vi "Main.vi"(10 "Mensajes Sub panel":refnum<vi>, 11 "Module Admin":refnum<class "Delacor_lib_QMH_Module Admin.lvclass">) -> ()   [LabVIEW 2019, in "Analisis.lvlib"]
doc: "This template is based off of the Queued Message Handler design pattern and the Queued Message Handler project template that ships with LabVIEW.\n\nThe main difference is that the queue is private to this module and communication between modules is performed via Broadcast and Request events.\n\nRequest events are wrapped in public API methods and are handled in the Event Handling Loop (EHL) of this VI. Any module can register for Broadcast events sent by this module. The EHL generates messages based on user interface actions.\n\nThe Message Handling Loop (MHL) processes messages generated by the EHL, or by other messages. The messages are string values, so new messages can be added easily to the Message Cases case structure in the MHL. Each message cluster can also provide an optional value for Message Data, which is a variant that can be converted to whatever message-specific data is required.\n_____\nBased on Delacor QMH Project Template 5.0.0.82.\n\nAnalisis\n\nEste modulo es similar a el de adquisicion y base de datos, solamente que aqui ciclamos el analisis de la imagen por medio de un VI generado desde vission assistant, en el cual analisamos, la forma de una marca, el color de la tarjeta y el nombre del indivduo, al igual que los otros modulos cuenta con un helper loop y eventos de configuracion."
uses:
  Analisis.lvlib
  <vilib>/Delacor/Delacor QMH/Libraries/Module Admin_class/Delacor_lib_QMH_Module Admin.lvclass
  Module Data--cluster.ctl
  Iniciar analisis Argument--cluster.ctl
  Parar Analisis Argument--cluster.ctl
  <vilib>/vision/Image Controls.llb/IMAQ Image.ctl
  Analisis de imagenes Argument--cluster.ctl
  Stop Argument--cluster.ctl
  <vilib>/Delacor/Delacor QMH/Libraries/Message Queue_class/Delacor_lib_QMH_Message Queue.lvclass/Delacor_lib_QMH_Message Queue.ctl
  <vilib>/Delacor/Delacor QMH/Libraries/Module Admin_class/Delacor_lib_QMH_Module Admin.lvclass/Delacor_lib_QMH_Module Admin.ctl
  <vilib>/Utility/miscctls.llb/LVPointTypeDef.ctl
  <vilib>/Delacor/Delacor QMH/Libraries/Message Queue_class/Delacor_lib_QMH_Enqueue Message (Single).vi
  <vilib>/Delacor/Delacor QMH/Libraries/Module Admin_class/Delacor_lib_QMH_Get External Launch.vi
  <vilib>/Utility/error.llb/Error Cluster From Error Code.vi
  <vilib>/ErrorRing/Error Ring.xnode
  <vilib>/Delacor/Delacor QMH/Libraries/Message Queue_class/Delacor_lib_QMH_Message Queue.lvclass
  Base de datos/Base de datos.lvlib
panel:
  out "Hora de Entrada":timestamp
  out "Area":string
  out "Nombre":string
  out "Empresa":string
  out "error out":errorcluster
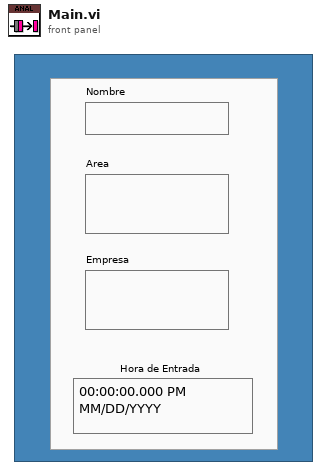
[diagram p1: front panel]
types:
  T1 = typedef "Analisis.lvlib/Request Events--cluster.ctl" = cluster{"Stop Module":refnum<user-event>, "Show Panel":refnum<user-event>, "Hide Panel":refnum<user-event>, "Get Module Execution Status":refnum<user-event>, "Show Diagram":refnum<user-event>, "Iniciar analisis":refnum<user-event>, "Parar Analisis":refnum<user-event>, "Analisis de imagenes":refnum<user-event>}
  T2 = typedef "Analisis.lvlib/Module Data--cluster.ctl" = cluster{"Status":string}
  T3 = typedef "IMAQ Image.ctl" = refnum<image>
  T4 = typedef "Analisis.lvlib/Parar Analisis Argument--cluster.ctl" = cluster{"Boolean":bool}
  T5 = typedef "Analisis.lvlib/Analisis de imagenes Argument--cluster.ctl" = cluster{"New Image":T3}
  T6 = enum32{"invalid lock state", "Not Locked", "Locked (No Password)", "Password-protected"}
  T7 = typedef "Analisis.lvlib/Stop Argument--cluster.ctl" = cluster{"Origin":string, "Exit via Stop Module Req?":bool, "Wait for Module to stop?":bool}
  T8 = typedef "LVPointTypeDef.ctl" = cluster{"Horizontal":i16, "Vertical":i16}
  T9 = enum32{"Invalid", "Standard", "Closed", "Hidden", "Minimized", "Maximized"}
  T10 = typedef "Image Type" = u32
  T11 = typedef "Analisis.lvlib/Iniciar analisis Argument--cluster.ctl" = cluster{"Boolean":bool}
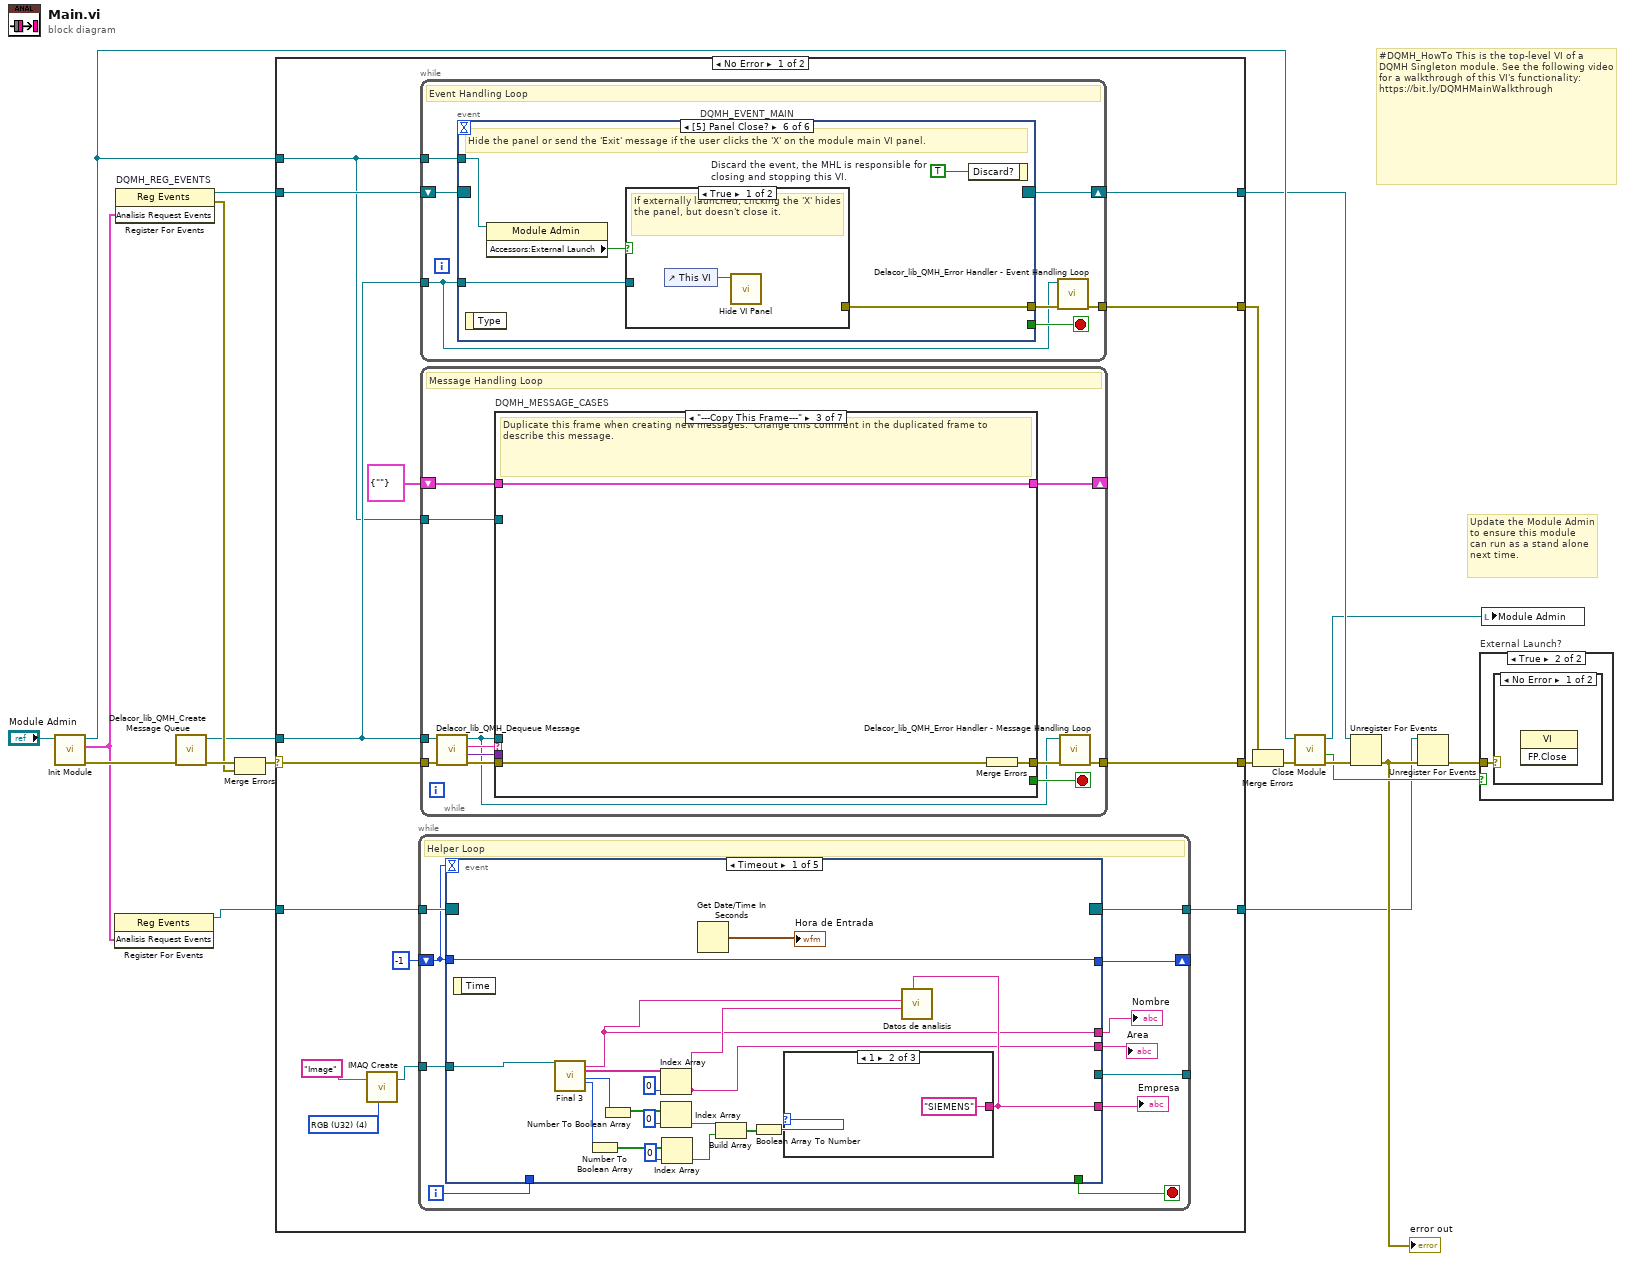
[diagram p0: block diagram]
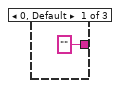
[diagram p2: hidden frame]
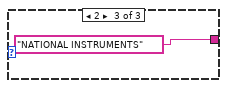
[diagram p3: hidden frame]
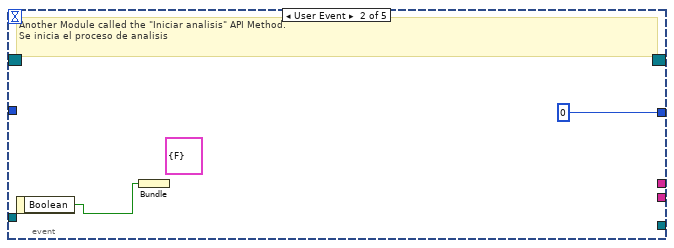
[diagram p4: hidden frame]
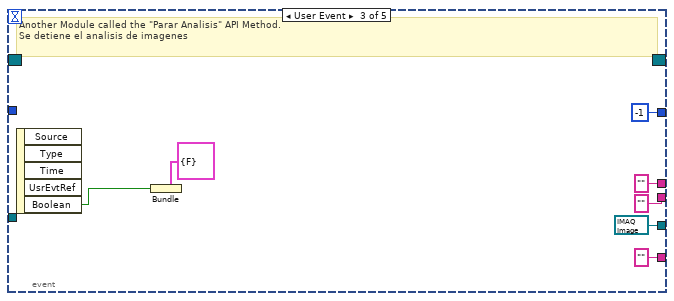
[diagram p5: hidden frame]
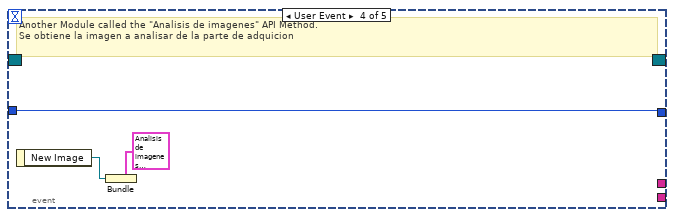
[diagram p6: hidden frame]
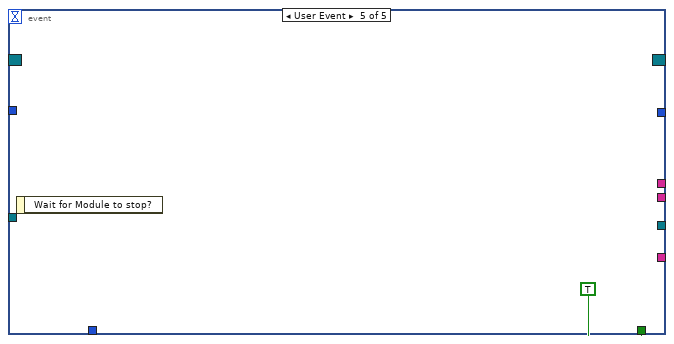
[diagram p7: hidden frame]
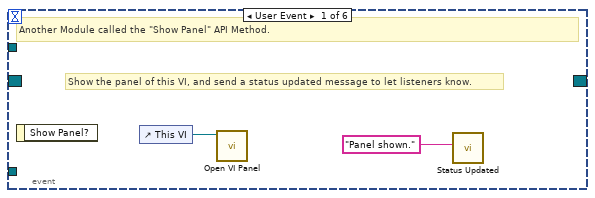
[diagram p8: hidden frame]
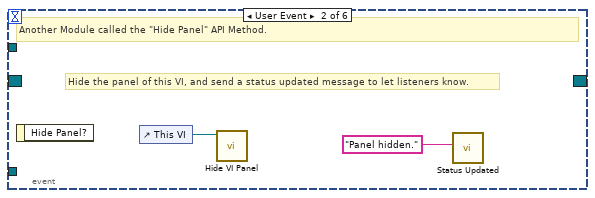
[diagram p9: hidden frame]
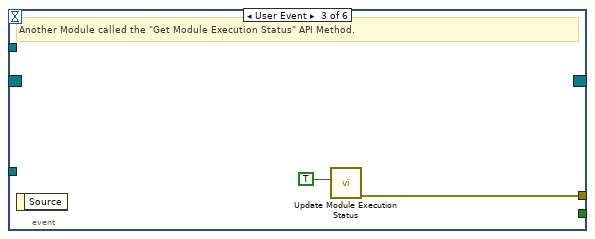
[diagram p10: hidden frame]
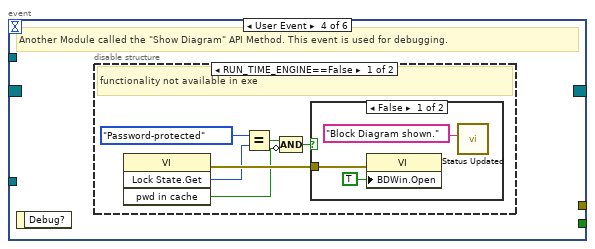
[diagram p11: hidden frame]
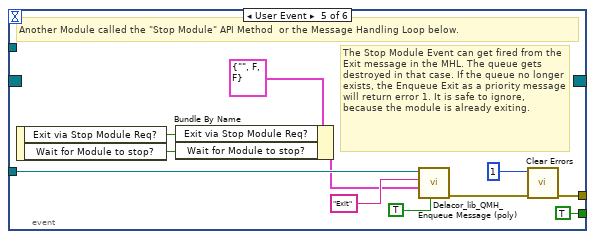
[diagram p14: hidden frame]
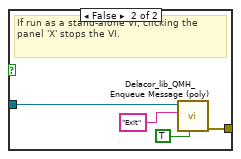
[diagram p15: hidden frame]
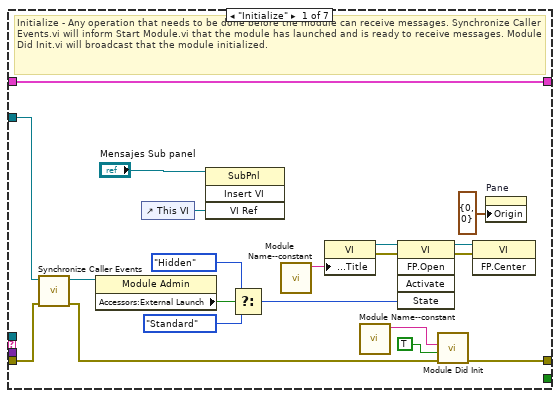
[diagram p16: hidden frame]
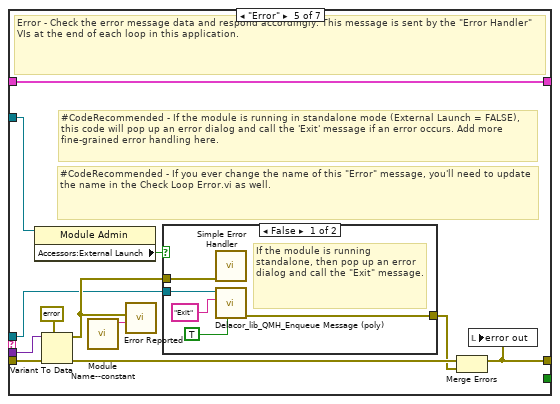
[diagram p19: hidden frame]
diagram:
  # "#DQMH_HowTo This is the top-level VI of a DQMH Singleton module. See the following video for a walkthrough of this VI's functionality: https://bit.ly/DQMHMainWalkthrough"
  # "Update the Module Admin to ensure this module can run as a stand alone next time."
  n1 = call "Init Module.vi"("Singleton Module Admin in"="Module Admin") -> ("error out"=w19:errorcluster, "Analisis Request Events"=w5:T1, "Singleton Module Admin out"=w12:refnum<class "Delacor_lib_QMH_Module Admin.lvclass">)  [unwired: 8 in]
  n2 = register-events(w5) -> (reference out=w4:refnum<event-registration>)  [unwired: 2 in, 1 out]
  n3 = register-events "DQMH_REG_EVENTS"(w5) -> (reference out=w10:refnum<event-registration>, error out=w13:errorcluster)  [unwired: 2 in]
  n4 = call <vilib>:"Delacor_lib_QMH_Create Message Queue.vi"("error in (no error)"=w19) -> ("error out"=w15:errorcluster, "Message Queue"=w9:refnum<class "Delacor_lib_QMH_Message Queue.lvclass">)  [unwired: 9 in]
  n5 = Merge Errors(w15, w13) -> (w14:errorcluster)
  n6 = case shown="No Error" w14 {
    selector: w14 -> [w32 w211]
    tunnel: [w34 w210] -> w20
    tunnel: [w31 w216] -> w11
    tunnel: w10 -> [w29 w216]
    tunnel: w9 -> [w28 w209]
    tunnel: [w33 _] -> w17
    tunnel: w12 -> [w27 w212]
    tunnel: w4 -> [w26 w208]
    tunnel: [w25 w208] -> w1
    frame No Error {
      w22 = T10 4 items=["Grayscale (U8)", "Grayscale (I16)", "Grayscale (SGL)", "Complex (CSG)", "RGB (U32)", "HSL (U32)", "RGB (U64)", "Grayscale (U16)"] ("Image Type")
      n7 = call "IMAQ Create"("Image Name"="Image", "Image Type"=w22) -> ("New Image"=w21:T3)  [unwired: 3 in, 1 out]
      n8 = while {
        tunnel: w26 -> [w45]
        tunnel: [w44] -> w25
        shift-right: [w42] -> _
        shift-left: -1 -> [w41]
        tunnel: [w40] -> _
        tunnel: w21 -> [w39]
        i -> [w38]
        stop <- w43 stop-if-true
        # "Helper Loop"
        n9 = event shown="[0] Timeout" {
          selector: w45 -> [_ _ _ _ _]
          dyn-events: [_ _ _ _ _] -> w44
          timeout: w41 -> [_ _ _ _ _]
          tunnel: [_ _ _ _ TRUE] -> w43
          tunnel: [w63 0 -1 w76 _] -> w42
          tunnel: w41 -> [w63 _ _ w76 _]
          tunnel: [_ _ T3 refnum ("New Image") _ _] -> w40
          tunnel: w39 -> [w62 _ _ _ _]
          tunnel: w38 -> [_ _ _ _ _]
          tunnel: [w49 _ "" ("String 4") _ _] -> w35
          tunnel: [w48 _ "" ("Class") _ _] -> w36
          tunnel: [w47 _ "" ("String (OCR/OCV 1)") _ _] -> w37
          event Timeout {
            n10 = event-data() -> ()  [unwired: 1 in, 1 out]
            n11 = call "Final 3.vi"("Image In"=w62) -> ("String (OCR/OCV 1)"=w47:string, "Classes (Color Classification 1)"=w61:string[], "Number of Matches (Color Location 1)"=w59:i32, "Number of Matches (Color Location 2)"=w58:i32)  [unwired: 20 in, 3 out]
            n12 = Number To Boolean Array(number=w58) -> (Boolean array=w54:bool[])
            n13 = Number To Boolean Array(number=w59) -> (Boolean array=w55:bool[])
            n14 = Index Array(array=w61, index=0) -> (element=w48:string)
            n15 = Index Array(array=w55, index=0) -> (element=w53:bool)
            n16 = Index Array(array=w54, index=0) -> (element=w52:bool)
            n17 = Get Date/Time In Seconds() -> (seconds since 1Jan1904=→"Hora de Entrada":timestamp)
            n18 = Build Array(w53, w52) -> (w51:bool[])
            n19 = Boolean Array To Number(Boolean array=w51) -> (number=w50:u32)
            n20 = case shown="1" w50 {
              tunnel: ["" ("String 4") "SIEMENS" ("String 4") "NATIONAL INSTRUMENTS" ("String 4")] -> w49
              frame 0, Default {
              }
              frame 1 {
              }
              frame 2 {
              }
            }
            n21 = call "Datos de analisis.vi"("String 3"=w49, "String 2"=w48, "String"=w47) -> ()  [unwired: 8 in, 1 out]
          }
          event User Event {
            (unwired) T11 {"Boolean"=FALSE} ("Iniciar analisis Argument")
            # "Another Module called the \"Iniciar analisis\" API Method.\nSe inicia el proceso de analisis"
            n22 = event-data() -> ("Boolean"=w68:bool)  [unwired: 1 in]
            n23 = Bundle("Boolean"=w68) -> ()  [unwired: 1 in, 1 out]
          }
          event User Event {
            # "Another Module called the \"Parar Analisis\" API Method.\nSe detiene el analisis de imagenes"
            n24 = event-data() -> ("Boolean"=w74:bool)  [unwired: 1 in, 4 out]
            n25 = Bundle(cluster=T4 {"Boolean"=FALSE} ("Parar Analisis Argument"), "Boolean"=w74) -> ()  [unwired: 1 out]
          }
          event User Event {
            # "Another Module called the \"Analisis de imagenes\" API Method.\nSe obtiene la imagen a analisar de la parte de adquicion"
            n26 = event-data() -> ("New Image"=w77:T3)  [unwired: 1 in]
            n27 = Bundle(cluster=T5 {"New Image"=refnum} ("Analisis de imagenes Argument"), "New Image"=w77) -> ()  [unwired: 1 out]
          }
          event User Event {
            n28 = event-data() -> ()  [unwired: 1 in, 1 out]
          }
        }
        "Area" <- w36
        "Nombre" <- w37
        "Empresa" <- w35
      }
      n29 = while {
        tunnel: w28 -> [w80]
        shift-right: [w83] -> w31
        shift-left: w29 -> [w84]
        tunnel: [w85] -> w33
        tunnel: w27 -> [w81]
        stop <- w82 stop-if-true
        # "Event Handling Loop"
        n30 = event "DQMH_EVENT_MAIN" shown="[5] Panel Close?" {
          selector: w84 -> [_ _ _ _ _ _]
          dyn-events: [_ _ _ _ _ _] -> w83
          timeout: _ -> [_ _ _ _ _ _]
          tunnel: [_ _ _ _ TRUE ("Discard?") _] -> w82
          tunnel: w80 -> [_ _ _ _ w108 w115]
          tunnel: [_ _ w92 _ w111 w117] -> w86
          tunnel: w81 -> [_ _ _ _ _ w114]
          event User Event {
            # "Show the panel of this VI, and send a status updated message to let listeners know."
            # "Another Module called the \"Show Panel\" API Method."
            n31 = event-data() -> ()  [unwired: 1 in, 1 out]
            n32 = control-ref of="This VI"() -> (w88:refnum<vi>)
            n33 = call "Open VI Panel.vi"("VI"=w88) -> ()  [unwired: 10 in, 1 out]
            n34 = call "Status Updated.vi"("Status"="Panel shown." ("format string")) -> ()  [unwired: 10 in, 1 out]
          }
          event User Event {
            # "Hide the panel of this VI, and send a status updated message to let listeners know."
            # "Another Module called the \"Hide Panel\" API Method."
            n35 = event-data() -> ()  [unwired: 1 in, 1 out]
            n36 = control-ref of="This VI"() -> (w90:refnum<vi>)
            n37 = call "Hide VI Panel.vi"("VI"=w90) -> ()  [unwired: 10 in, 1 out]
            n38 = call "Status Updated.vi"("Status"="Panel hidden." ("format string")) -> ()  [unwired: 10 in, 1 out]
          }
          event User Event {
            # "Another Module called the \"Get Module Execution Status\" API Method."
            n39 = event-data() -> ()  [unwired: 1 in, 1 out]
            n40 = call "Update Module Execution Status.vi"("Running?"=TRUE) -> ("error out"=w92:errorcluster)  [unwired: 10 in]
          }
          event User Event {
            # "Another Module called the \"Show Diagram\" API Method. This event is used for debugging."
            n41 = event-data() -> ()  [unwired: 1 in, 1 out]
            n42 = disable-structure shown="RUN_TIME_ENGINE==False" {
              frame condition #0 (active) {
                # "functionality not available in exe"
                n43 = invoke class="VI" method="Lock State.Get"() -> (error out=w98:errorcluster, "Get Lock State"=w97:T6, "pwd in cache"=w94:bool)  [unwired: 4 in, 1 out]
                n44 = Equal?(x=T6."Password-protected", y=w97) -> (x = y?=w95:bool)
                n45 = Compound Arithmetic op=AND(w95, invert w94) -> (w93:bool)
                n46 = case shown="False" w93 {
                  tunnel: w98 -> [w101 _]
                  frame False {
                    n47 = property class="VI"(error in=w101, "BDWin.Open"=TRUE ("Block Diagram Window:Open")) -> ()  [unwired: 1 in, 2 out]
                    n48 = call "Status Updated.vi"("Status"="Block Diagram shown." ("format string")) -> ()  [unwired: 10 in, 1 out]
                  }
                  frame True {
                    # "Password-protected VI, and the password is not in the cache. Do not show the diagram."
                  }
                }
              }
              frame condition #1 {
              }
            }
          }
          event User Event {
            # "The Stop Module Event can get fired from the Exit message in the MHL. The queue gets destroyed in that case. If the queue no longer exists, the Enqueue Exit as a priority message will return error 1. It is safe to ignore, because the module is already exiting."
            # "Another Module called the \"Stop Module\" API Method  or the Message Handling Loop below."
            n49 = event-data() -> ("Exit via Stop Module Req?"=w104:bool, "Wait for Module to stop?"=w103:bool)  [unwired: 1 in]
            n50 = Bundle By Name(cluster=T7 {"Origin"="", "Exit via Stop Module Req?"=FALSE, "Wait for Module to stop?"=FALSE} ("Stop Argument"), "Exit via Stop Module Req?"=w104, "Wait for Module to stop?"=w103) -> (w102:T7)
            n51 = call-poly <vilib>:"Delacor_lib_QMH_Enqueue Message (poly).vi"("Priority Message? (F)"=TRUE, "Message Data"=w102, "Message"="Exit", "Message Queue in"=w108) -> ("error out"=w112:errorcluster)  [unwired: 6 in, 1 out]
            n52 = call <vilib>:"Clear Errors.vi"("error in (no error)"=w112, "specific error code to clear (0: all)"=1) -> ("error out"=w111:errorcluster)  [unwired: 4 in, 1 out]
          }
          event Panel Close? {
            w116 = TRUE  # Discard the event, the MHL is responsible for closing and stopping this VI.
            # "Hide the panel or send the 'Exit' message if the user clicks the 'X' on the module main VI panel."
            n53 = event-data() -> ()  [unwired: 1 in, 1 out]
            n54 = property class="Module Admin"(reference=w114) -> ("Accessors:External Launch"=w113:bool)  [unwired: 1 in, 2 out]
            n55 = case shown="True" w113 {
              tunnel: w115 -> [_ w121]
              tunnel: [_ w122] -> w117
              frame True {
                # "If externally launched, clicking the 'X' hides the panel, but doesn't close it."
                n56 = control-ref of="This VI"() -> (w118:refnum<vi>)
                n57 = call "Hide VI Panel.vi"("VI"=w118) -> ()  [unwired: 10 in, 1 out]
              }
              frame False {
                # "If run as a stand-alone VI, clicking the panel 'X' stops the VI."
                n58 = call-poly <vilib>:"Delacor_lib_QMH_Enqueue Message (poly).vi"("Priority Message? (F)"=TRUE, "Message"="Exit", "Message Queue in"=w121) -> ("error out"=w122:errorcluster)  [unwired: 7 in, 1 out]
              }
            }
            n59 = event-data("Discard?"=w116) -> ()  [unwired: 1 in, 1 out]
          }
        }
        n60 = call-dynamic "Delacor_lib_QMH_Error Handler - Event Handling Loop.vi"("error in (no error)"=w86, "Message Queue in"=w80) -> ("dup error in"=w85:errorcluster)  [unwired: 8 in, 1 out]
      }
      n61 = while {
        tunnel: w28 -> [w125]
        shift-right: [w129] -> _
        shift-left: T2 {"Status"=""} ("Data Cluster") -> [w130]
        tunnel: w32 -> [w133]
        tunnel: [w131] -> w34
        tunnel: w27 -> [w123]
        stop <- w128 stop-if-true
        # "Message Handling Loop"
        n62 = call-dynamic "Delacor_lib_QMH_Dequeue Message.vi"("error in (no error)"=w133, "Message Queue in"=w125) -> ("error out"=w132:errorcluster, "Message Data"=w126:variant, "Message"=w127:string, "Message Queue out"=w124:refnum<class "Delacor_lib_QMH_Message Queue.lvclass">)  [unwired: 6 in]
        n63 = case "DQMH_MESSAGE_CASES" shown="\"---Copy This Frame---\"" w127 {
          selector: w127 -> [_ _ _ _ _ _ w195]
          tunnel: w124 -> [_ _ _ _ w165 w187 _]
          tunnel: w132 -> [w152 w156 w159 w161 w172 w193 w197]
          tunnel: [w150 w156 w158 w161 w168 w190 w198] -> w134
          tunnel: w130 -> [w141 w155 w157 w160 w167 w186 w196]
          tunnel: [w141 w155 w157 w160 w167 w186 w196] -> w129
          tunnel: [_ _ _ _ _ w185 _] -> w128
          tunnel: w126 -> [_ _ _ _ w166 w184 _]
          tunnel: w123 -> [w142 _ _ _ w164 w179 _]
          frame "Initialize" {
            # "Initialize - Any operation that needs to be done before the module can receive messages. Synchronize Caller Events.vi will inform Start Module.vi that the module has launched and is ready to receive messages. Module Did Init.vi will broadcast that the module initialized."
            n64 = call "Synchronize Caller Events.vi"("error in (no error)"=w152, "Singleton Module Admin in"=w142) -> ("error out"=w151:errorcluster, "Singleton Module Admin out"=w138:refnum<class "Delacor_lib_QMH_Module Admin.lvclass">)  [unwired: 8 in]
            n65 = property class="Module Admin"(reference=w138) -> ("Accessors:External Launch"=w146:bool)  [unwired: 1 in, 2 out]
            n66 = control-ref of="This VI"() -> (w135:refnum<vi>)
            n67 = invoke class="SubPnl" method="Insert VI"(reference="Mensajes Sub panel", "VI Ref"=w135) -> ()  [unwired: 2 in, 4 out]
            n68 = Select(t=T9."Hidden" ("State"), s=w146, f=T9."Standard" ("State")) -> (s? t:f=w143:T9)
            n69 = call "Module Name--constant.vi"() -> ("Module Name"=w149:string)  [unwired: 11 in]
            n70 = property class="VI"("Front Panel.Title"=w149) -> (reference out=w148:refnum<vi>, error out=w154:errorcluster)  [unwired: 2 in]
            n71 = call "Module Name--constant.vi"() -> ("Module Name"=w139:string)  [unwired: 11 in]
            n72 = invoke class="VI" method="FP.Open"(reference=w148, error in=w154, "State"=w143) -> (reference out=w147:refnum<vi>, error out=w153:errorcluster)  [unwired: 2 in, 3 out]
            n73 = call "Module Did Init.vi"("error in (no error)"=w151, "Initialized?"=TRUE, "Origin"=w139) -> ("error out"=w150:errorcluster)  [unwired: 8 in]
            n74 = invoke class="VI" method="FP.Center"(reference=w147, error in=w153) -> ()  [unwired: 1 in, 3 out]
            n75 = property on="Pane" class="Pane"("Origin"=T8 {"Horizontal"=0, "Vertical"=0}) -> ()  [unwired: 2 in, 2 out]
          }
          frame "--- Module Specific ---" {
            # "Separator -- The following cases handle messages specific to this Module."
          }
          frame "---Copy This Frame---" {
            # "Duplicate this frame when creating new messages.  Change this comment in the duplicated frame to describe this message."
            n76 = Merge Errors(w159) -> (w158:errorcluster)
          }
          frame "--- Exit and Error Handling---" {
            # "Separator - The following cases handle errors and exit messages."
          }
          frame "Error" {
            # "#CodeRecommended - If you ever change the name of this \"Error\" message, you'll need to update the name in the Check Loop Error.vi as well."
            # "#CodeRecommended - If the module is running in standalone mode (External Launch = FALSE), this code will pop up an error dialog and call the 'Exit' message if an error occurs. Add more fine-grained error handling here."
            # "Error - Check the error message data and respond accordingly. This message is sent by the \"Error Handler\" VIs at the end of each loop in this application."
            n77 = property class="Module Admin"(reference=w164) -> ("Accessors:External Launch"=w163:bool)  [unwired: 1 in, 2 out]
            n78 = Variant To Data(error in=w172, type=errorcluster {"status"=FALSE, "code"=0, "source"=""} ("error constant"), Variant=w166) -> (data=w173:errorcluster, error out=w170:errorcluster)
            n79 = call "Module Name--constant.vi"() -> ("Module Name"=w162:string)  [unwired: 11 in]
            n80 = call "Error Reported.vi"("Additional Information"=w162, "Error"=w173) -> ()  [unwired: 9 in, 1 out]
            n81 = case shown="False" w163 {
              tunnel: [w178 _] -> w169
              tunnel: w165 -> [w176 _]
              tunnel: w173 -> [w177 _]
              frame False {
                # "If the module is running standalone, then pop up an error dialog and call the \"Exit\" message."
                n82 = call <vilib>:"Simple Error Handler.vi"("error in (no error)"=w177) -> ()  [unwired: 4 in, 5 out]
                n83 = call-poly <vilib>:"Delacor_lib_QMH_Enqueue Message (poly).vi"("Priority Message? (F)"=TRUE, "Message"="Exit", "Message Queue in"=w176) -> ("error out"=w178:errorcluster)  [unwired: 7 in, 1 out]
              }
              frame True {
                # "If the module was launched externally, calling the Error Reported broadcast VI is the only action performed by the \"Error\" message. The module's caller can then process the error appropriately."
              }
            }
            n84 = Merge Errors(w170, w169) -> (w168:errorcluster)
            n85 = local write "error out"(w168) -> ()
          }
          frame "Exit" {
            w183 = 91  # 91: not all Exit messages will have an argument
            w185 = TRUE  # Stop the VI
            # "Release the message queue reference"
            # "#CodeNeeded - Add any required cleanup code here"
            # "Exit - Exit the application."
            n86 = Variant To Data(error in=w193, type=T7 {"Origin"="", "Exit via Stop Module Req?"=FALSE, "Wait for Module to stop?"=FALSE} ("Stop Argument"), Variant=w184) -> (data=w181:T7, error out=w189:errorcluster)
            n87 = call <vilib>:"Clear Errors.vi"("error in (no error)"=w189, "specific error code to clear (0: all)"=w183) -> ("error out"=w192:errorcluster)  [unwired: 4 in, 1 out]
            n88 = control-ref of="This VI"() -> (w180:refnum<vi>)
            n89 = call-dynamic "Delacor_lib_QMH_Release Message Queue.vi"("error in (no error)"=w192, "Message Queue"=w187) -> ("error out"=w191:errorcluster)  [unwired: 9 in]
            n90 = call "Handle Exit.vi"("Stop Argument"=w181, "Admin in"=w179, "VI reference"=w180) -> ("error out"=w188:errorcluster)  [unwired: 7 in, 1 out]
            n91 = Merge Errors(w191, w188) -> (w190:errorcluster)
          }
          frame Default {
            # "'Default' case only runs if there is a message that isn't defined in any of the other cases.  Output a programming error."
            n92 = call "Module Name--constant.vi"() -> ("Module Name"=w194:string)  [unwired: 11 in]
            n93 = xnode "Error Ring"("parameter 0"=w195, "parameter 1"=w194) -> ("error out"=w199:errorcluster)
            n94 = Merge Errors(w197, w199) -> (w198:errorcluster)
          }
        }
        n95 = call-dynamic "Delacor_lib_QMH_Error Handler - Message Handling Loop.vi"("error in (no error)"=w134, "Message Queue in"=w124) -> ("dup error in"=w131:errorcluster)  [unwired: 8 in, 1 out]
      }
    }
    frame Error {
      # "Synchronize Caller Events.vi will inform Start Module.vi that the module has launched and will let the code calling Start Module.vi register for broadcasts and would permit the caller receive the broadcast that an error occurred at launch time."
      n96 = call-dynamic "Delacor_lib_QMH_Release Message Queue.vi"("error in (no error)"=w211, "Message Queue"=w209) -> ("error out"=w210:errorcluster)  [unwired: 9 in]
      n97 = call "Synchronize Caller Events.vi"("Singleton Module Admin in"=w212) -> ("error out"=w217:errorcluster)  [unwired: 9 in, 1 out]
      n98 = call "Module Name--constant.vi"() -> ("Module Name"=w215:string)  [unwired: 11 in]
      n99 = Format Into String(format string="An error occurred during initialization. %s is no longer running.", w215) -> (resulting string=w213:string)  [unwired: 2 in, 1 out]
      n100 = Merge Errors(w210, w217) -> (w218:errorcluster)
      n101 = call "Error Reported.vi"("Additional Information"=w213, "Error"=w218) -> ()  [unwired: 9 in, 1 out]
    }
  }
  n102 = Merge Errors(w17, w20) -> (w16:errorcluster)
  n103 = call "Close Module.vi"("error in (no error)"=w16, "Module Admin in"=w12) -> ("error out"=w18:errorcluster, "External Launch"=w6:bool, "Module Admin out"=w7:refnum<class "Delacor_lib_QMH_Module Admin.lvclass">)  [unwired: 7 in]
  n104 = Unregister For Events(event registration refnum=w11, error in=w18) -> (error out=w2:errorcluster)
  "error out" <- w2
  n105 = Unregister For Events(event registration refnum=w1, error in=w2) -> (error out=w3:errorcluster)
  n106 = case "External Launch?" shown="True" w6 {
    tunnel: w3 -> [_ w219]
    frame False {
    }
    frame True {
      n107 = case shown="No Error" w219 {
        frame No Error {
          n108 = invoke class="VI" method="FP.Close"() -> ()  [unwired: 3 in, 3 out]
        }
        frame Error {
          n109 = invoke class="VI" method="FP.Open"("Activate"=TRUE ("Activate?")) -> ()  [unwired: 4 in, 5 out]
        }
      }
    }
  }
  n110 = local write "Module Admin"(w7) -> ()
